vi "Overlay Track.vi"(8 "error in (no error)":errorcluster, 10 "Flattened Image":T1, 11 "Track":T2={"Tip 1"={"Point"={"X"=0.0, "Y"=0.0}, "Angle"=0.0, "Frame Number"=0, "ROI Descriptor"={"Global Rectangle"=[], "Contours"=[]}, "Curvature"=0.0, "Label"="Non-tip"}, "Tip 2"={"Point"={"X"=0.0, "Y"=0.0}, "Angle"=0.0, "Frame Number"=0, "ROI Descriptor"={"Global Rectangle"=[], "Contours"=[]}, "Curvature"=0.0, "Label"="Non-tip"}, "Label"="", "ROI Descriptor"={"Global Rectangle"=[], "Contours"=[]}} {"ROI Descriptor"."Contours"."Type" items=["No Selection", "Point", "Line", "Rectangle", "Oval", "Polygon", "Freehand Region", "Annulus", "Unused2", "Unused3", "Broken Line", "Freehand Line", "Rotated Rectangle"]; "Tip 2"."ROI Descriptor"."Contours"."Type" items=["No Selection", "Point", "Line", "Rectangle", "Oval", "Polygon", "Freehand Region", "Annulus", "Unused2", "Unused3", "Broken Line", "Freehand Line", "Rotated Rectangle"]; "Tip 2"."Point"."Y" format="%.2f"; "Tip 2"."Point"."X" format="%.2f"; "Tip 1"."ROI Descriptor"."Contours"."Type" items=["No Selection", "Point", "Line", "Rectangle", "Oval", "Polygon", "Freehand Region", "Annulus", "Unused2", "Unused3", "Broken Line", "Freehand Line", "Rotated Rectangle"]; "Tip 1"."Point"."Y" format="%.2f"; "Tip 1"."Point"."X" format="%.2f"}) -> (0 "error out":errorcluster, 3 "Image out":T1)   [LabVIEW 2013]
uses:
  Controls/Track.ctl
  Controls/Tip.ctl
  <vilib>/vision/Image Controls.llb/IMAQ Image.ctl
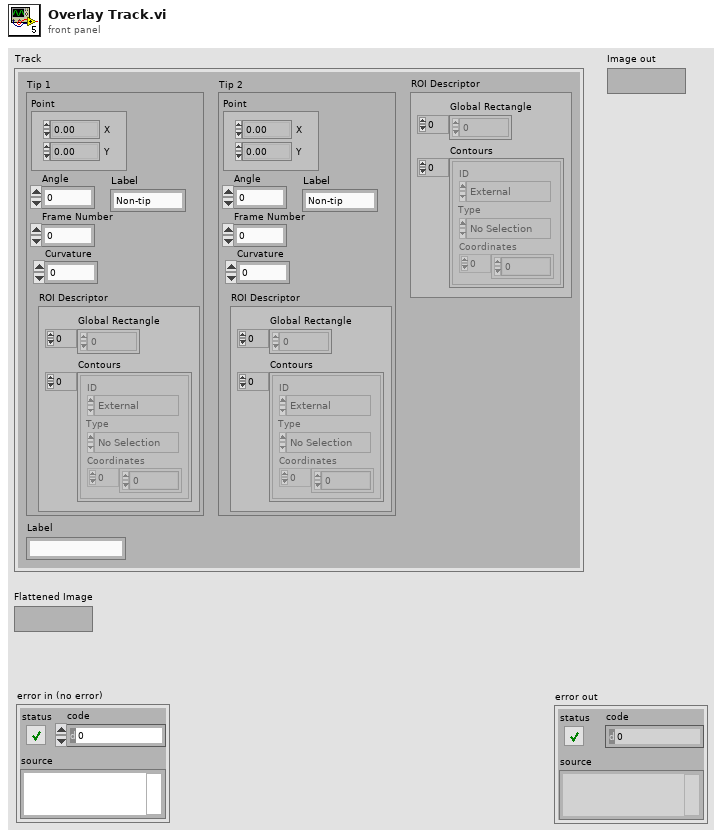
[diagram p1: front panel]
types:
  T1 = typedef "IMAQ Image.ctl" = refnum<image>
  T2 = typedef "Track.ctl" = cluster{"Tip 1":T3, "Tip 2":T3, "Label":string, "ROI Descriptor":T5}
  T3 = typedef "Tip.ctl" = cluster{"Point":T4, "Angle":dbl, "Frame Number":i32, "ROI Descriptor":T5, "Curvature":dbl, "Label":string}
  T4 = typedef "IMAQ Point" = cluster{"X":sgl, "Y":sgl}
  T5 = typedef "ROI Descriptor" = cluster{"Global Rectangle":i32[], "Contours":cluster{"ID":enum32{"External", "Internal"}, "Type":u32, "Coordinates":i32[]}[]}
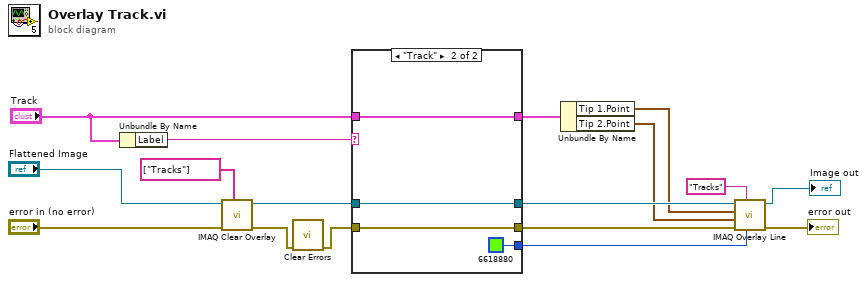
[diagram p0: block diagram]
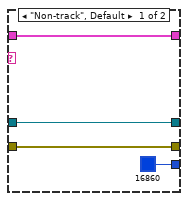
[diagram p2: hidden frame]
diagram:
  n1 = Unbundle By Name("Track") -> ("Label"=w17:string)
  n2 = call "IMAQ Clear Overlay"("Groups"=string[] ["Tracks"], "error in (no error)"="error in (no error)", "Image"="Flattened Image") -> ("error out"=w2:errorcluster, "Image Out"=w12:T1)  [unwired: 7 in]
  n3 = call <vilib>:"Clear Errors.vi"("error in (no error)"=w2) -> ("error out"=w1:errorcluster)  [unwired: 6 in]
  n4 = case shown="\"Track\"" w17 {
    tunnel: "Track" -> [w19 w25]
    tunnel: [w19 w25] -> w11
    tunnel: w12 -> [w21 w23]
    tunnel: [w20 w24] -> w9
    tunnel: w1 -> [w20 w24]
    tunnel: [w21 w23] -> w10
    tunnel: [u32 16860 u32 6618880] -> w5
    frame "Non-track", Default {
    }
    frame "Track" {
    }
  }
  n5 = Unbundle By Name(w11) -> ("Tip 1.Point"=w8:T4, "Tip 2.Point"=w7:T4)
  n6 = call "IMAQ Overlay Line"("Color"=w5, "Group"="Tracks", "error in (no error)"=w9, "End Point"=w7, "Start Point"=w8, "Image"=w10) -> ("error out"=→"error out":errorcluster, "Image Out"=→"Image out":T1)  [unwired: 4 in]
